vi "仪器初始化proto.vi"() -> ()   [LabVIEW 2017]
doc: "使用该模板构建标准状态机设计模式。各状态执行代码并决定转移状态。将该设计模式与根据用户动作响应而执行代码的用户界面事件处理器模式相比较。同时将该设计模式与每段消息处理代码可以将零至多个新消息加入队列的队列消息处理器模式相比较。\n注：该模板的设计未遵守最新NI推荐的编程风格。请通过“创建项目”对话框（而不要采用该模板），创建基于项目的标准状态机模式的完整实现。"
uses:
  labview setup procedure.ctl
  device index.ctl
panel:
  out "error out":errorcluster caption="错误输出"
  in  "error in (no error)":errorcluster caption="错误输入（无错误）"
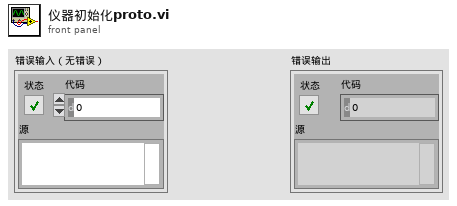
[diagram p1: front panel]
types:
  T1 = typedef "device index.ctl" = cluster{"Position no.":i32, "Rotaion no.":i32, "piezo no.":i32, "mg position":dbl, "mg rotation":dbl, "piezo position":dbl, "pos axes":string[], "rot axes":string[], "piezo axes":string[]}
  T2 = typedef "labview setup procedure.ctl" = enum16{"仪器注销", "注册并校准仪器", "完成设置", "清除ROI", "结束磁铁循环"}
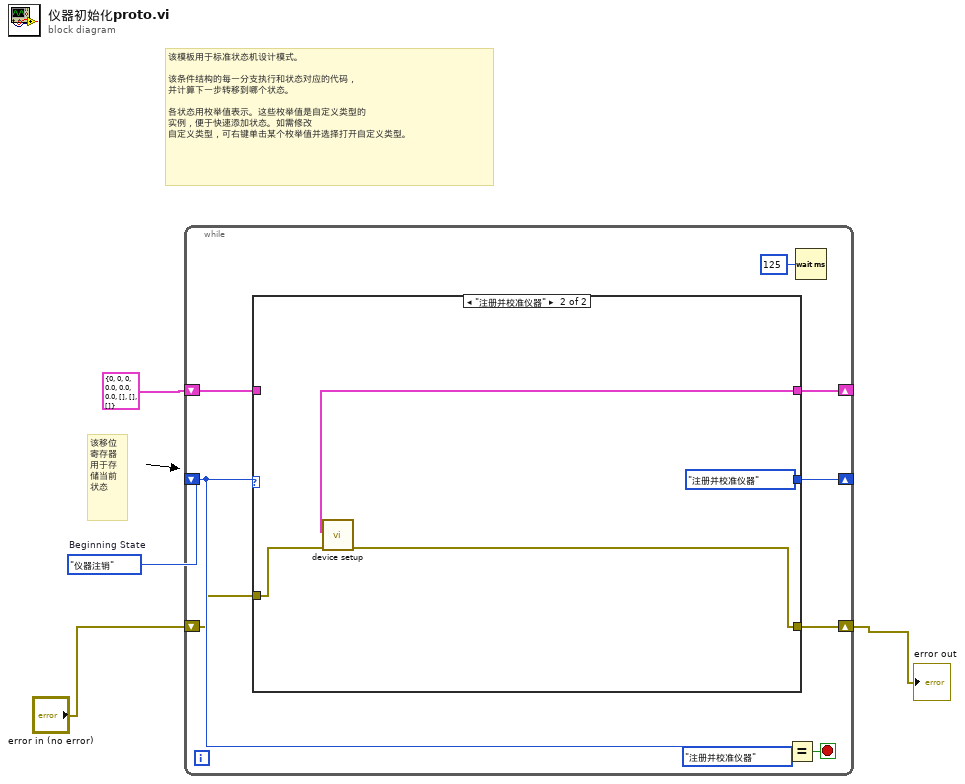
[diagram p0: block diagram]
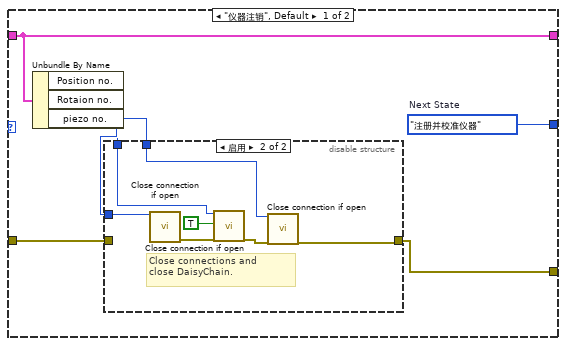
[diagram p2: hidden frame]
diagram:
  w4 = labview_setup_procedure."仪器注销"  # Beginning State
  # "该模板用于标准状态机设计模式。\n\n该条件结构的每一分支执行和状态对应的代码，\n并计算下一步转移到哪个状态。\n\n各状态用枚举值表示。这些枚举值是自定义类型的\n实例，便于快速添加状态。如需修改\n自定义类型，可右键单击某个枚举值并选择打开自定义类型。"
  # "该移位\n寄存器\n用于存\n储当前\n状态"
  n1 = while {
    shift-right: [w10] -> _
    shift-left: w4 -> [w11]
    shift-right: [w5] -> _
    shift-left: T1 {"Position no."=0, "Rotaion no."=0, "piezo no."=0, "mg position"=0.0, "mg rotation"=0.0, "piezo position"=0.0, "pos axes"=[], "rot axes"=[], "piezo axes"=[]} ("device index") -> [w8]
    shift-right: [w6] -> w1
    shift-left: "error in (no error)" -> [w7]
    stop <- w13 stop-if-true
    n2 = case shown="\"注册并校准仪器\"" w11 {
      tunnel: [w20 labview_setup_procedure."注册并校准仪器" ("Next State")] -> w10
      tunnel: w8 -> [w14 _]
      tunnel: w7 -> [w16 w31]
      tunnel: [w15 w30] -> w6
      tunnel: [w14 w29] -> w5
      frame "仪器注销", Default {
        w20 = labview_setup_procedure."注册并校准仪器"  # Next State
        n3 = Unbundle By Name(w14) -> ("Position no."=w19:i32, "Rotaion no."=w18:i32, "piezo no."=w17:i32)
        n4 = disable-structure shown="启用" {
          disable-tunnel: w19 -> [_ w25]
          disable-tunnel: w18 -> [_ w24]
          disable-tunnel: w17 -> [_ w23]
          disable-tunnel: w16 -> [w21 _]
          disable-tunnel: [w21 w22] -> w15
          frame Disabled {
          }
          frame Enabled {
            # "Close connections and\nclose DaisyChain."
            n5 = call "Close connection if open.vi"("System no."=w25) -> ("error out"=w26:errorcluster)  [unwired: 17 in, 1 out]
            n6 = call "Close connection if open.vi"("System no."=w24, "Close DaisyChain"=TRUE, "error in"=w26) -> ("error out"=w28:errorcluster)  [unwired: 15 in, 1 out]
            n7 = call "Close connection if open.vi"("System no."=w23, "error in"=w28) -> ("error out"=w22:errorcluster)  [unwired: 16 in, 1 out]
          }
        }
      }
      frame "注册并校准仪器" {
        n8 = call "device setup.vi"("error in (no error)"=w31) -> ("error out"=w30:errorcluster, "device index out"=w29:T1)  [unwired: 9 in]
      }
    }
    n9 = Equal?(x=w11, y=labview_setup_procedure."注册并校准仪器" ("States")) -> (x = y?=w13:bool)
    n10 = Wait (ms)(milliseconds to wait=u32 125) -> ()  [unwired: 1 out]
  }
  "error out" <- w1
